vi "process data.vi"(0 "Frequency (Hz)":dbl=128.0, 2 "Reference Signal":i32, 5 "sensor input":dbl[][](array[numeric])=array52386x3[157158 elements], 7 "In Signals":dbl[][](array[numeric]), 9 "FFT interval (s)":dbl=4.0, 11 "Normalize":bool, 12 "End time (s)":dbl=42.75184275184275) -> (1 "Fundamental frequency":dbl(slide) scale=0.0..10.0, 3 "FFT":T1, 4 "peaks":dbl[][](array[numeric]), 6 "Magnitude of time data":cluster{dbl[], dbl[]}, 8 "x',y',z'":T2, 10 "Signals":dbl[][](array[numeric]), 13 "correlation array":dbl[](array[numeric]), 14 "Filtered signal":dbl[](graph), 15 "Primary and secondary axis power":dbl[](array[slide]) scale=0.0..800.0)   [LabVIEW 2009]
panel:
  out "Matched signal":dynamicdata(graph)
  out "max correlation Secondary":dbl(slide) scale=0.0..1.0
  out "max correlation Primary":dbl(slide) scale=0.0..1.0
  out "max amplitude":dbl(slide) scale=0.0..6.0
  out "peak big":dbl[](array[numeric])
  out "peak med":dbl[](array[numeric])
  out "peak small":dbl[](array[numeric])
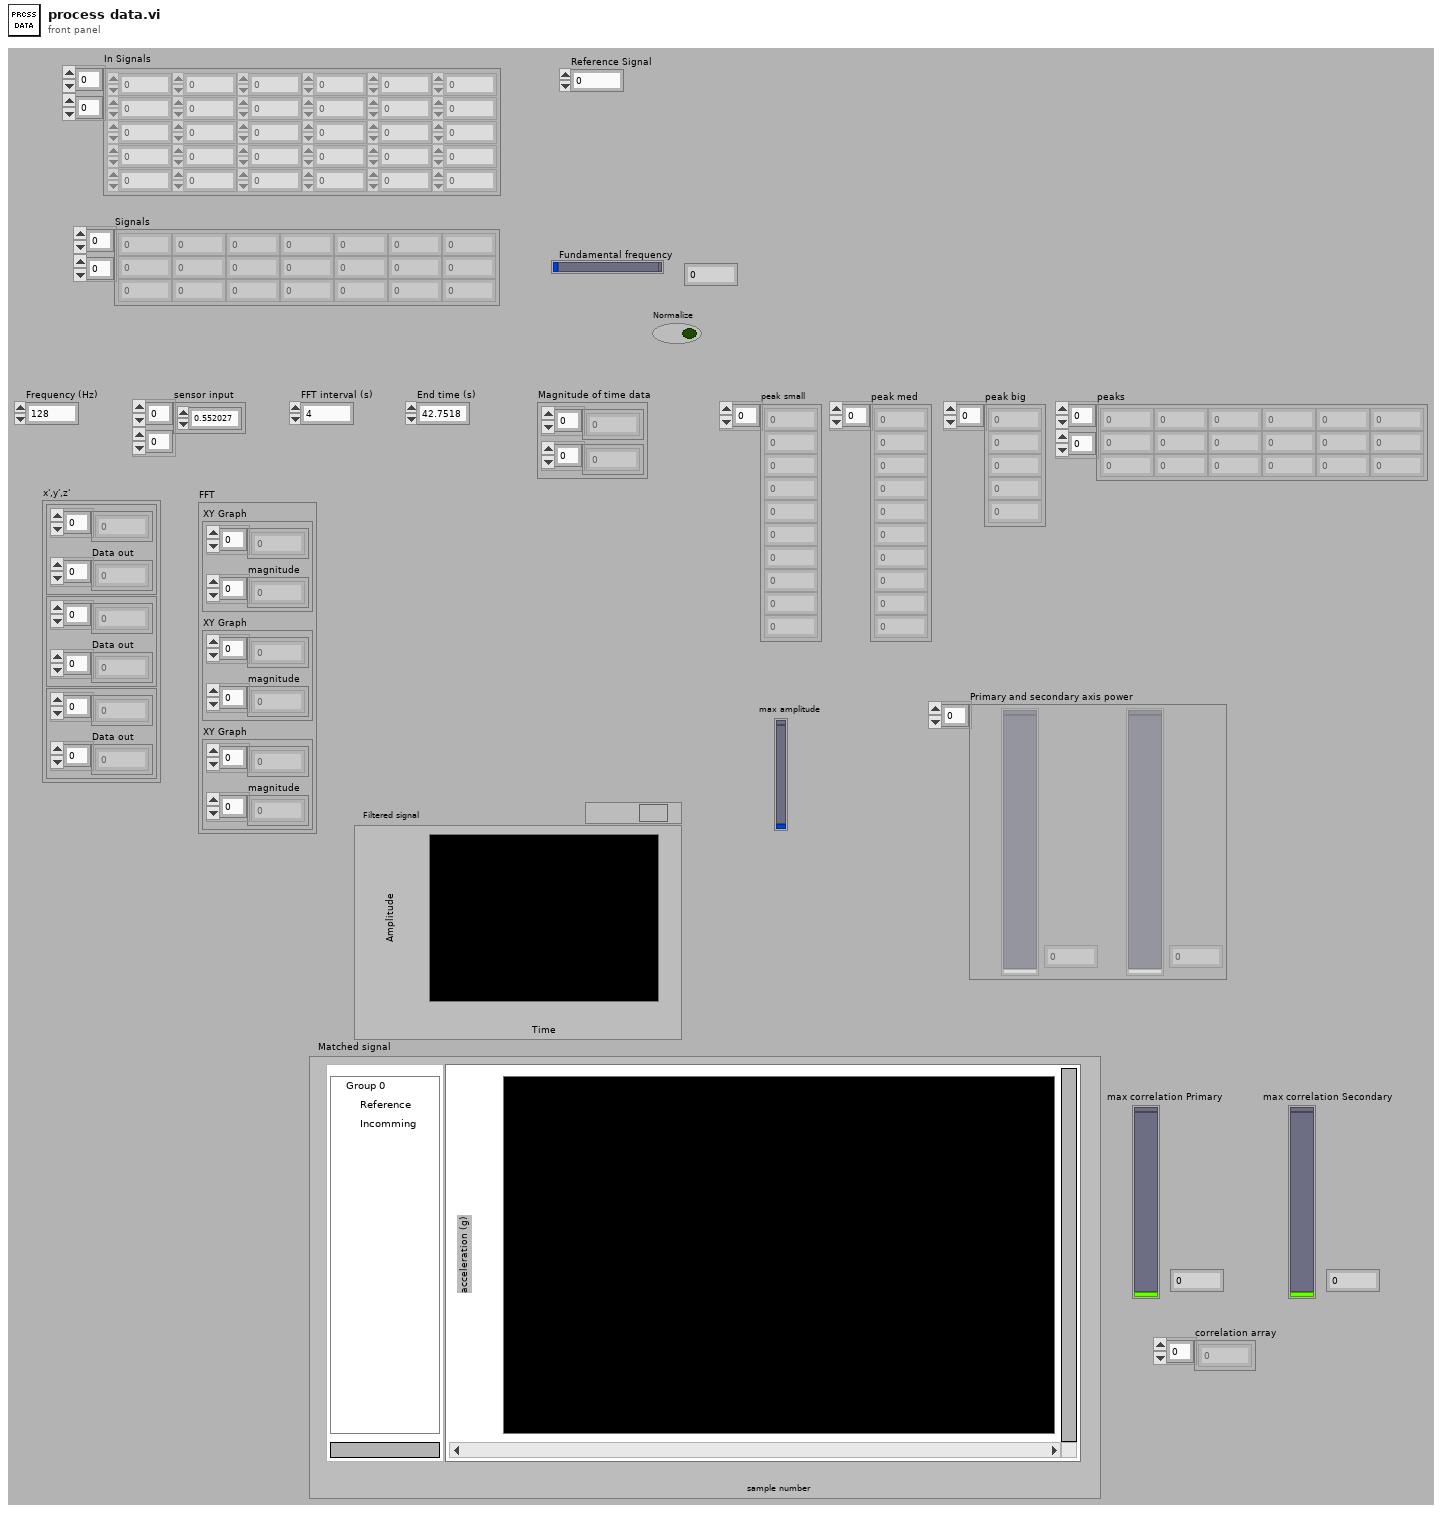
[diagram p1: front panel]
types:
  T1 = cluster{"XY Graph":cluster{dbl[], "magnitude":dbl[]}, "XY Graph":cluster{dbl[], "magnitude":dbl[]}, "XY Graph":cluster{dbl[], "magnitude":dbl[]}}
  T2 = cluster{cluster{dbl[], "Data out":dbl[]}, cluster{dbl[], "Data out":dbl[]}, cluster{dbl[], "Data out":dbl[]}}
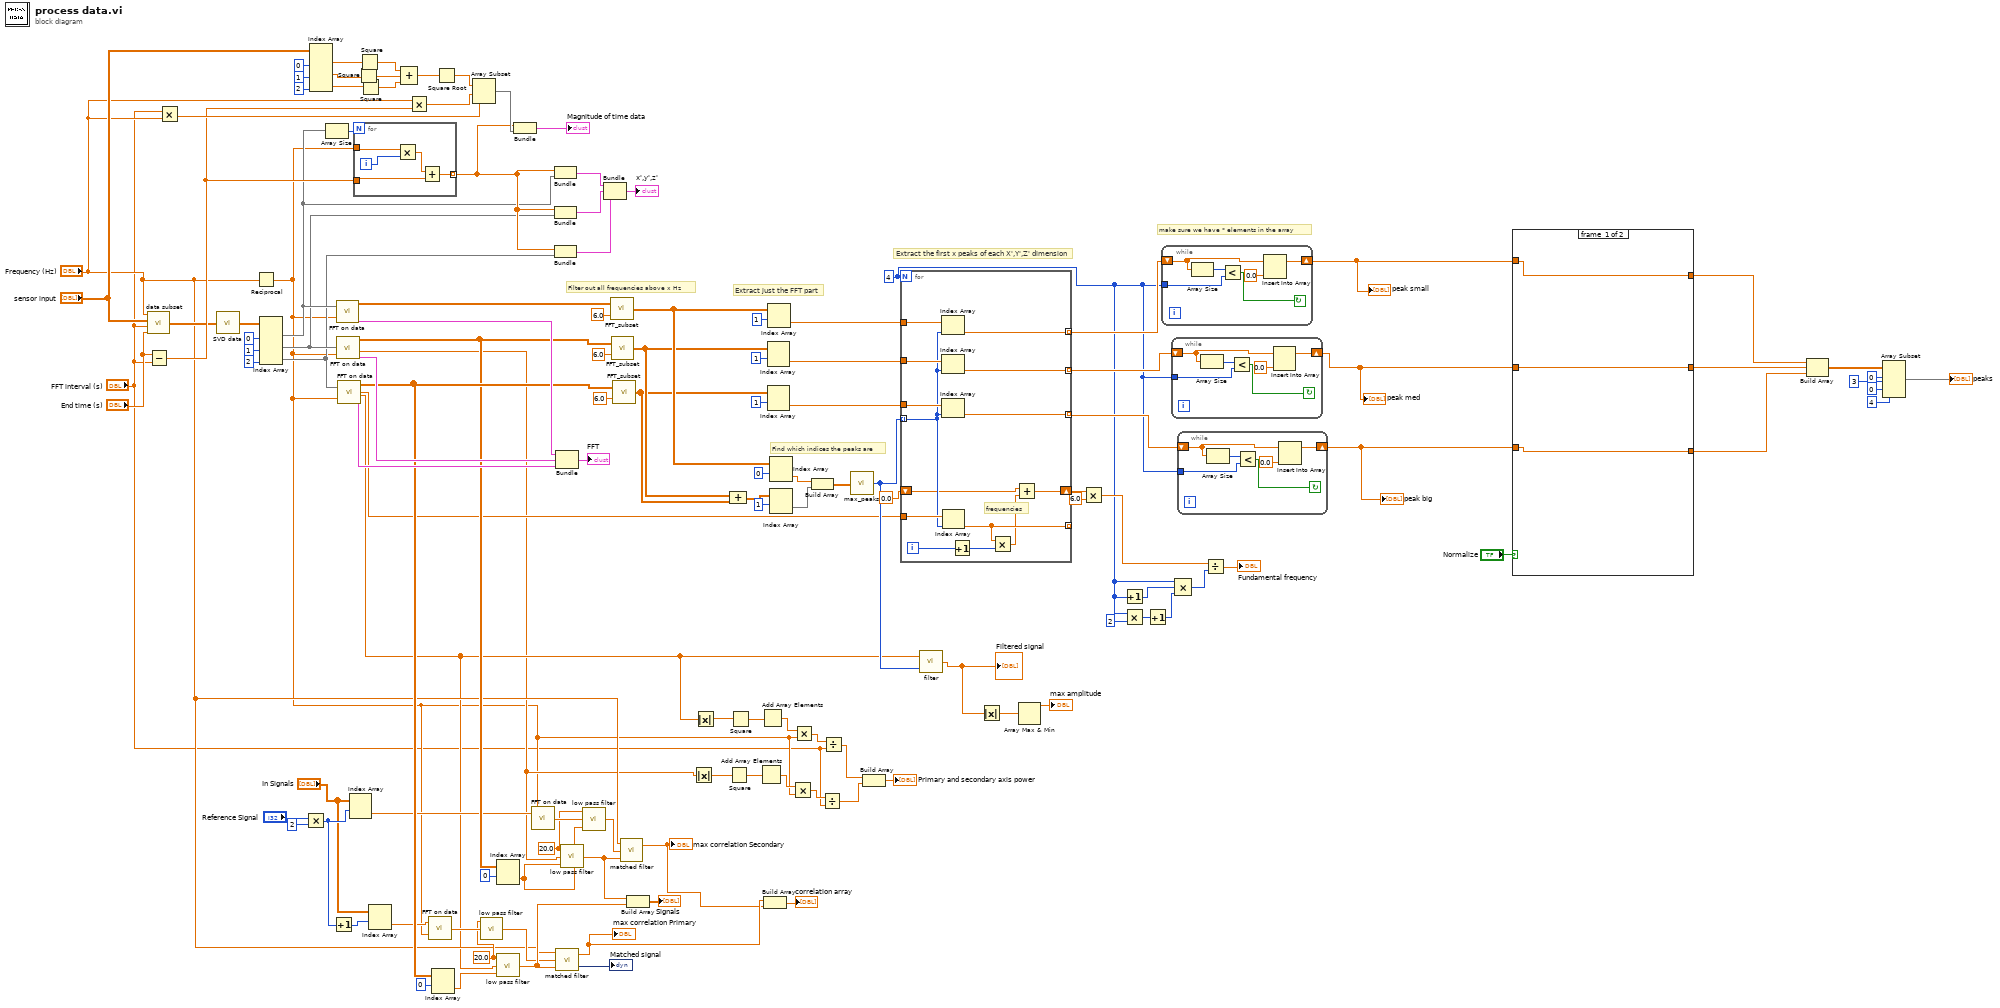
[diagram p0: block diagram]
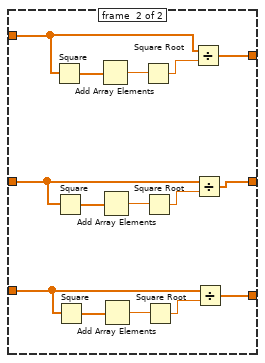
[diagram p2: hidden frame]
diagram:
  w22 = 20.0 ("cut off frequency")
  w18 = 20.0 ("cut off frequency")
  w56 = 4
  # "make sure we have * elements in the array"
  # "Extract the first x peaks of each X',Y',Z' dimension"
  # "Find which indices the peaks are"
  # "Filter out all frequencies above x Hz"
  # "Extract just the FFT part"
  n1 = call "data subset.vi"("End time (s)"="End time (s)", "FFT interval (s)"="FFT interval (s)", "sensor"="sensor input", "Frequency (Hz)"="Frequency (Hz)") -> ("sensor subset"=w30:dbl[][])
  n2 = Subtract(x="End time (s)", y="FFT interval (s)") -> (x-y=w124:dbl)
  n3 = Multiply(x="FFT interval (s)", y="Frequency (Hz)") -> (x*y=w128:dbl)
  n4 = call "SVD data.vi"("Data"=w30) -> ("Data out"=w102:dbl[][])
  n5 = Reciprocal(x="Frequency (Hz)") -> (1/x=w5:dbl)
  n6 = Index Array(array=w102, index (col) #1=0 ("disabled index (col)"), index (col) #2=1 ("index (col)"), index (col) #3=2 ("index (col)")) -> (element #1=w71:dbl[], element #2=w70:dbl[], element #3=w31:dbl[])  [unwired: 3 in]
  n7 = Multiply(x="Reference Signal", y=2) -> (x*y=w36:i32)
  n8 = Index Array(array="sensor input", index (col) #1=0 ("disabled index (col)"), index (col) #2=1 ("index (col)"), index (col) #3=2 ("index (col)")) -> (element #1=w115:dbl[], element #2=w114:dbl[], element #3=w116:dbl[])  [unwired: 3 in]
  n9 = Array Size(array=w71) -> (size(s)=w106:i32)
  n10 = Increment(x=w36) -> (x+1=w34:i32)
  n11 = call "FFT on data.vi"("dt"=w5, "Data"=w71) -> ("XY Graph"=w98:cluster{dbl[], "magnitude":dbl[]}, "output"=w46:dbl[][])  [unwired: 3 out]
  n12 = call "FFT on data.vi"("dt"=w5, "Data"=w70) -> ("XY Graph"=w97:cluster{dbl[], "magnitude":dbl[]}, "FFT {X}"=w6:cdb[], "output"=w32:dbl[][])  [unwired: 2 out]
  n13 = call "FFT on data.vi"("dt"=w5, "Data"=w31) -> ("XY Graph"=w121:cluster{dbl[], "magnitude":dbl[]}, "FFT {X}"=w15:cdb[], "output"=w43:dbl[][], "frequency (Hz)"=w16:dbl[])  [unwired: 1 out]
  n14 = Index Array(array="In Signals", index (row)=w36) -> (element=w26:dbl[])  [unwired: 1 in]
  n15 = for {
    N: w106 -> [_]
    tunnel: w5 -> [w134]
    tunnel: w124 -> [w132]
    tunnel: [w130] -> w122 mode=indexing
    i -> [w133]
    n16 = Multiply(x=w134, y=w133) -> (x*y=w131:dbl)
    n17 = Add(x=w131, y=w132) -> (x+y=w130:dbl)
  }
  n18 = Square(x=w114) -> (x^2=w118:dbl[])
  n19 = Square(x=w115) -> (x^2=w117:dbl[])
  n20 = Square(x=w116) -> (x^2=w119:dbl[])
  n21 = Index Array(array="In Signals", index (row)=w34) -> (element=w20:dbl[])  [unwired: 1 in]
  n22 = Compound Arithmetic op=ADD(w117, w118, w119) -> (w120:dbl[])
  n23 = Multiply(x="Frequency (Hz)", y=w124) -> (x*y=w125:dbl)
  n24 = call "FFT on data.vi"("dt"=w5, "Data"=w20) -> ("FFT {X}"=w21:cdb[])  [unwired: 4 out]
  n25 = Index Array(array=w43, index (row)=0 ("disabled index (col)")) -> (element=w45:dbl[])  [unwired: 1 in]
  n26 = Square Root(x=w120) -> (sqrt(x)=w126:dbl[])
  n27 = Array Subset(array=w126, index=w125, length=w128) -> (w127:dbl[])
  n28 = call "low pass filter.vi"("input FFT"=w21, "cut off frequency"=w18) -> ("Output Time Domain"=w19:dbl[])  [unwired: 1 in]
  n29 = Index Array(array=w32, index (row)=0 ("disabled index (col)")) -> (element=w24:dbl[])  [unwired: 1 in]
  n30 = call "low pass filter.vi"("Input frequencies"=w45, "input FFT"=w15, "cut off frequency"=w18) -> ("Output Time Domain"=w40:dbl[])
  n31 = Bundle(w122, w127) -> (→"Magnitude of time data":cluster{dbl[], dbl[]})  [unwired: 1 in]
  n32 = call "FFT on data.vi"("dt"=w5, "Data"=w26) -> ("FFT {X}"=w25:cdb[])  [unwired: 4 out]
  n33 = Bundle(w122, "Data out"=w71) -> (w108:cluster{dbl[], "Data out":dbl[]})  [unwired: 1 in]
  n34 = Bundle(w122, "Data out"=w70) -> (w109:cluster{dbl[], "Data out":dbl[]})  [unwired: 1 in]
  n35 = Bundle(w122, "Data out"=w31) -> (w110:cluster{dbl[], "Data out":dbl[]})  [unwired: 1 in]
  n36 = Bundle("XY Graph"=w98, "XY Graph"=w97, "XY Graph"=w121) -> (→"FFT":T1)  [unwired: 1 in]
  n37 = call "matched filter.vi"("incoming signal"=w40, "reference signal"=w19, "Sampling Frq"="Frequency (Hz)") -> ("Matched signal"=→"Matched signal":dynamicdata, "max correlation"=w29:dbl)
  "max correlation Primary" <- w29
  n38 = call "low pass filter.vi"("Input frequencies"=w24, "input FFT"=w6, "cut off frequency"=w22) -> ("Output Time Domain"=w41:dbl[])
  n39 = call "low pass filter.vi"("Input frequencies"=w24, "input FFT"=w25, "cut off frequency"=w22) -> ("Output Time Domain"=w23:dbl[])
  n40 = Bundle(w108, w109, w110) -> (→"x',y',z'":T2)  [unwired: 1 in]
  n41 = call "FFT_subset.vi"("Hz"=6.0, "input"=w46) -> ("subarray"=w91:dbl[][])
  n42 = call "FFT_subset.vi"("Hz"=6.0, "input"=w32) -> ("subarray"=w88:dbl[][])
  n43 = call "FFT_subset.vi"("Hz"=6.0, "input"=w43) -> ("subarray"=w86:dbl[][])
  n44 = call "matched filter.vi"("incoming signal"=w41, "reference signal"=w23, "Sampling Frq"="Frequency (Hz)") -> ("max correlation"=w28:dbl)  [unwired: 1 out]
  "max correlation Secondary" <- w28
  n45 = Build Array(w41, w40) -> (→"Signals":dbl[][])
  n46 = Absolute Value(x=w6) -> (abs(x)=w10:dbl[])
  n47 = Absolute Value(x=w15) -> (abs(x)=w14:dbl[])
  n48 = Square(x=w10) -> (x^2=w9:dbl[])
  n49 = Square(x=w14) -> (x^2=w13:dbl[])
  n50 = Compound Arithmetic op=ADD(w88, w86) -> (w96:dbl[][])
  n51 = Add Array Elements(numeric array=w9) -> (sum=w8:dbl)
  n52 = Add Array Elements(numeric array=w13) -> (sum=w12:dbl)
  n53 = Build Array(w29, w28) -> (→"correlation array":dbl[])
  n54 = Index Array(array=w88, index (row)=1) -> (element=w84:dbl[])  [unwired: 1 in]
  n55 = Index Array(array=w86, index (row)=1) -> (element=w83:dbl[])  [unwired: 1 in]
  n56 = Index Array(array=w91, index (row)=1) -> (element=w89:dbl[])  [unwired: 1 in]
  n57 = Index Array(array=w91, index (row)=0) -> (element=w94:dbl[])  [unwired: 1 in]
  n58 = Index Array(array=w96, index (row)=1) -> (element=w93:dbl[])  [unwired: 1 in]
  n59 = Multiply(x=w8, y=w5) -> (x*y=w7:dbl)
  n60 = Multiply(x=w12, y=w5) -> (x*y=w11:dbl)
  n61 = Build Array(w94, w93) -> (w92:dbl[][])
  n62 = Divide(x=w7, y="FFT interval (s)") -> (x/y=w2:dbl)
  n63 = Divide(x=w11, y="FFT interval (s)") -> (x/y=w3:dbl)
  n64 = call "max_peaks.vi"("FFT in"=w92) -> ("peak indices"=w51:i32[])
  n65 = Build Array(w3, w2) -> (→"Primary and secondary axis power":dbl[])
  n66 = for {
    N: w56 -> [_]
    tunnel: w51 -> [w141] mode=indexing
    tunnel: w89 -> [w148]
    tunnel: w84 -> [w147]
    tunnel: w83 -> [w146]
    tunnel: [w145] -> w80 mode=indexing
    tunnel: [w144] -> w79 mode=indexing
    tunnel: [w143] -> w78 mode=indexing
    tunnel: w16 -> [w142]
    tunnel: [w138] -> _ mode=indexing
    shift-right: [w135] -> w61
    shift-left: 0.0 -> [w136]
    i -> [w140]
    # "frequencies"
    n67 = Index Array(array=w148, index=w141) -> (element=w145:dbl)
    n68 = Index Array(array=w147, index=w141) -> (element=w144:dbl)
    n69 = Index Array(array=w146, index=w141) -> (element=w143:dbl)
    n70 = Index Array(array=w142, index=w141) -> (element=w138:dbl)
    n71 = Increment(x=w140) -> (x+1=w139:i32)
    n72 = Multiply(x=w138, y=w139) -> (x*y=w137:dbl)
    n73 = Add(x=w136, y=w137) -> (x+y=w135:dbl)
  }
  n74 = call "filter.vi"("peak indices"=w51, "FFT{x}"=w15) -> ("X"=w50:dbl[])
  "Filtered signal" <- w50
  n75 = Absolute Value(x=w50) -> (abs(x)=w49:dbl[])
  n76 = Array Max & Min(array=w49) -> (max value=→"max amplitude":dbl)  [unwired: 3 out]
  n77 = Multiply(x=w61, y=6.0) -> (x*y=w59:dbl)
  n78 = Increment(x=w56) -> (x+1=w55:i32)
  n79 = Multiply(x=w56, y=2) -> (x*y=w57:i32)
  n80 = Increment(x=w57) -> (x+1=w54:i32)
  n81 = while {
    tunnel: w56 -> [w153]
    shift-right: [w149] -> w63
    shift-left: w80 -> [w151]
    stop <- w152 continue-if-true
    n82 = Array Size(array=w151) -> (size(s)=w154:i32)
    n83 = Less?(x=w154, y=w153) -> (x < y?=w152:bool)
    n84 = Insert Into Array(array=w151, new element=0.0 ("new element/subarray")) -> (w149:dbl[])  [unwired: 1 in]
  }
  "peak small" <- w63
  n85 = while {
    tunnel: w56 -> [w159]
    shift-right: [w155] -> w67
    shift-left: w79 -> [w157]
    stop <- w158 continue-if-true
    n86 = Array Size(array=w157) -> (size(s)=w160:i32)
    n87 = Less?(x=w160, y=w159) -> (x < y?=w158:bool)
    n88 = Insert Into Array(array=w157, new element=0.0 ("new element/subarray")) -> (w155:dbl[])  [unwired: 1 in]
  }
  "peak med" <- w67
  n89 = Compound Arithmetic op=MULTIPLY(w56, w55, w54) -> (w53:i32)
  n90 = while {
    tunnel: w56 -> [w165]
    shift-right: [w161] -> w69
    shift-left: w78 -> [w163]
    stop <- w164 continue-if-true
    n91 = Array Size(array=w163) -> (size(s)=w166:i32)
    n92 = Less?(x=w166, y=w165) -> (x < y?=w164:bool)
    n93 = Insert Into Array(array=w163, new element=0.0 ("new element/subarray")) -> (w161:dbl[])  [unwired: 1 in]
  }
  "peak big" <- w69
  n94 = Divide(x=w59, y=w53) -> (x/y=→"Fundamental frequency":dbl)
  n95 = case shown="False" "Normalize" {
    tunnel: w69 -> [w167 w181]
    tunnel: [w167 w180] -> w68
    tunnel: w67 -> [w168 w173]
    tunnel: [w168 w172] -> w66
    tunnel: w63 -> [w169 w171]
    tunnel: [w169 w170] -> w65
    frame #0 {
    }
    frame #1 {
      n96 = Square(x=w171) -> (x^2=w177:dbl[])
      n97 = Square(x=w173) -> (x^2=w179:dbl[])
      n98 = Square(x=w181) -> (x^2=w184:dbl[])
      n99 = Add Array Elements(numeric array=w177) -> (sum=w176:dbl)
      n100 = Add Array Elements(numeric array=w179) -> (sum=w178:dbl)
      n101 = Add Array Elements(numeric array=w184) -> (sum=w183:dbl)
      n102 = Square Root(x=w176) -> (sqrt(x)=w175:dbl)
      n103 = Square Root(x=w178) -> (sqrt(x)=w174:dbl)
      n104 = Square Root(x=w183) -> (sqrt(x)=w182:dbl)
      n105 = Divide(x=w171, y=w175) -> (x/y=w170:dbl[])
      n106 = Divide(x=w173, y=w174) -> (x/y=w172:dbl[])
      n107 = Divide(x=w181, y=w182) -> (x/y=w180:dbl[])
    }
  }
  n108 = Build Array(w65, w66, w68) -> (w73:dbl[][])
  n109 = Array Subset(array=w73, index (row)=0 ("index"), length (row)=3 ("length"), index (col)=0 ("index"), length (col)=4 ("length")) -> (→"peaks":dbl[][])
